vi "Get_Transition_Points.vi"(0 "Analog_Waveform":waveform(dbl)(graph)={"t0"=timestamp(0 s since 1904-01-01), "dt"=1e-06, "Y"=array[5000 elements]}, 5 "Amplitude (V)":dbl=5.0) -> (4 "dt":dbl, 6 "Transition_Points":i32[](array[numeric]))   [LabVIEW 2023]
doc: "This VI gets the Transition points when the Analog waveform in given in."
uses:
  Controls/Index_Select.ctl
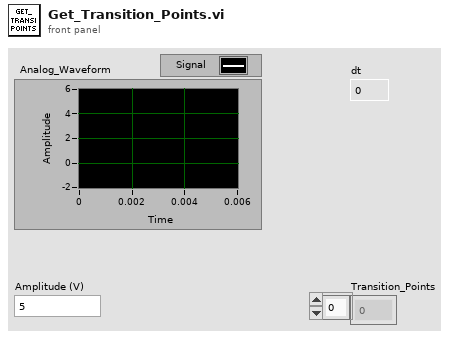
[diagram p1: front panel]
types:
  T1 = typedef "Index_Select.ctl" = enum16{"Wait_for_0", "Index_RTS", "Index_RTE", "Index_FTS", "Index_FTE"}
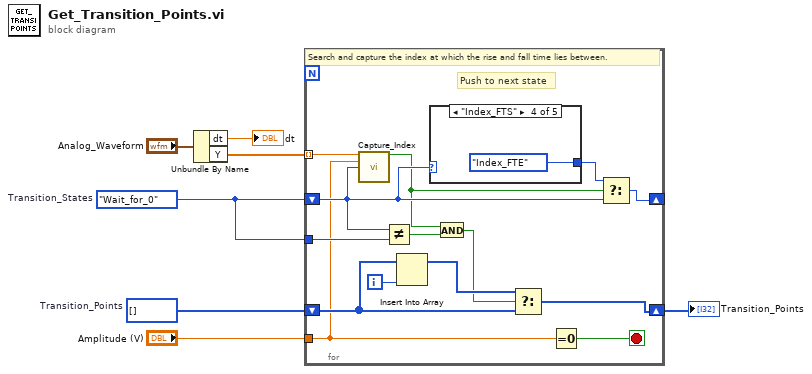
[diagram p0: block diagram]
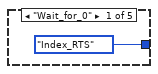
[diagram p2: hidden frame]
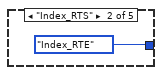
[diagram p3: hidden frame]
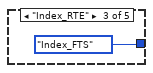
[diagram p4: hidden frame]
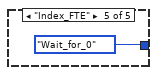
[diagram p5: hidden frame]
diagram:
  w4 = i32[] []  # Transition_Points
  w2 = Index_Select."Wait_for_0"  # Transition_States
  n1 = Unbundle By Name("Analog_Waveform") -> ("dt"=→"dt":dbl, "Y"=w6:dbl[])
  n2 = for {
    tunnel: w6 -> [w21] mode=indexing
    tunnel: "Amplitude (V)" -> [w9]
    shift-right: [w15] -> w3
    shift-left: w4 -> [w18]
    shift-right: [w17] -> _
    shift-left: w2 -> [w13]
    tunnel: w2 -> [w10]
    i -> [w20]
    stop <- w8 stop-if-true
    # "Push to next state"
    # "Search and capture the index at which the rise and fall time lies between."
    n3 = call "Capture_Index.vi"("Y"=w21, "Amplitude(V)"=w9, "Index_Select"=w13) -> ("Capture?"=w11:bool)  [unwired: 12 in]
    n4 = Not Equal?(x=w13, y=w10) -> (x != y?=w16:bool)
    n5 = Insert Into Array(array=w18, new element=w20) -> (w19:i32[])  [unwired: 1 in]
    n6 = case shown="\"Index_FTS\"" w13 {
      tunnel: [Index_Select."Index_RTS" Index_Select."Index_RTE" Index_Select."Index_FTS" Index_Select."Index_FTE" Index_Select."Wait_for_0"] -> w14
      frame "Wait_for_0" {
      }
      frame "Index_RTS" {
      }
      frame "Index_RTE" {
      }
      frame "Index_FTS" {
      }
      frame "Index_FTE" {
      }
    }
    n7 = And(x=w11, y=w16) -> (x .and. y?=w12:bool)
    n8 = Select(t=w19, s=w12, f=w18) -> (s? t:f=w15:i32[])
    n9 = Equal To 0?(x=w9) -> (x = 0?=w8:bool)
    n10 = Select(t=w14, s=w11, f=w13) -> (s? t:f=w17:T1)
  }
  "Transition_Points" <- w3
